vi "toString.vi"(8 "error in (no error)":errorcluster, 11 "MixerMessage in":refnum<class "MixerMessage.lvclass">) -> (0 "error out":errorcluster, 2 "String":string, 3 "MixerMessage out":refnum<class "MixerMessage.lvclass">)   [LabVIEW 2013, in "MixerMessage.lvclass"]
doc: "Format the message to a string. For each protocol that needs to be implemented. creata a child class of BaseMessage and overload this method"
uses:
  MixerMessage.lvclass
  MixerMessage.lvclass/MixerMessage.ctl
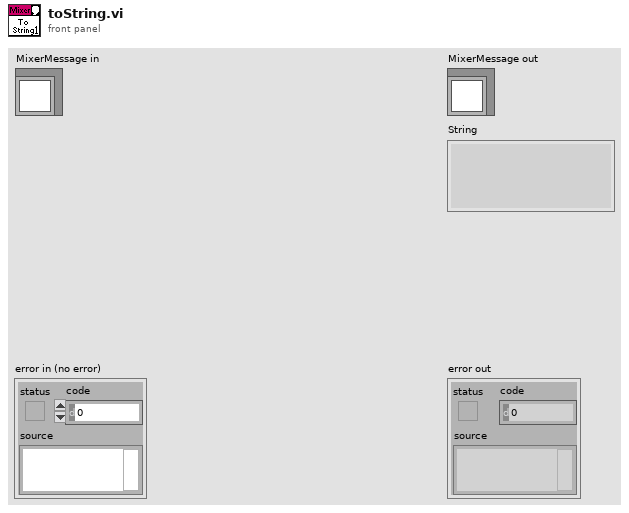
[diagram p1: front panel]
types:
  T1 = typedef "MixerMessage.lvclass/MixerOperation.ctl" = enum16{"Get", "Set"}
  T2 = typedef "MixerMessage.lvclass/MixerParam.ctl" = enum16{"a", "b", "fm", "delay", "delay delta"}
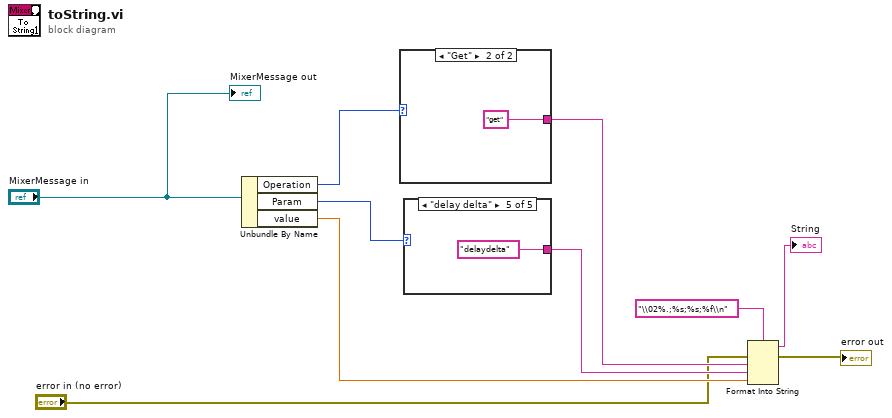
[diagram p0: block diagram]
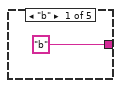
[diagram p2: hidden frame]
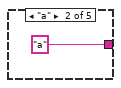
[diagram p3: hidden frame]
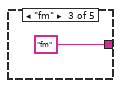
[diagram p4: hidden frame]
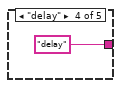
[diagram p5: hidden frame]
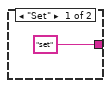
[diagram p6: hidden frame]
diagram:
  n1 = Unbundle By Name("MixerMessage in") -> ("Operation"=w10:T1, "Param"=w9:T2, "value"=w7:dbl)
  n2 = case shown="\"Get\"" w10 {
    tunnel: ["set" "get"] -> w5
    frame "Set" {
    }
    frame "Get" {
    }
  }
  n3 = case shown="\"delay delta\"" w9 {
    tunnel: ["b" "a" "fm" "delay" "delaydelta"] -> w6
    frame "b" {
    }
    frame "a" {
    }
    frame "fm" {
    }
    frame "delay" {
    }
    frame "delay delta" {
    }
  }
  n4 = Format Into String(format string="\\02%.;%s;%s;%f\\n", error in="error in (no error)", w5, w6, w7) -> (resulting string=→"String":string, error out=→"error out":errorcluster)  [unwired: 1 in]
  "MixerMessage out" <- "MixerMessage in"
